vi "image2slopes2phase.vi"(5 "Haso configuration file":path=path "C:/Program Files (x86)/Imagine Optic/Configuration Files/HASO3_first_7364.dat", 7 "Filter":u8[](array[numeric]), 8 "error in (no error)":errorcluster, 9 "Image in":refnum<class "Image.lvclass">, 10 "Phase in":refnum<class "Phase.lvclass">, 11 "HasoSlopes in":refnum<class "HasoSlopes.lvclass">) -> (0 "error out":errorcluster, 1 "Image out":refnum<class "Image.lvclass">, 2 "Phase out":refnum<class "Phase.lvclass">, 3 "HasoSlopes out":refnum<class "HasoSlopes.lvclass">)   [LabVIEW 2018]
uses:
  <userlib>/WaveKit.lib/Classes/Phase/Phase.lvclass
  <userlib>/WaveKit.lib/Controls/HasoSlopes.lvclass
  <userlib>/WaveKit.lib/Classes/Image/Image.lvclass
  <userlib>/WaveKit.lib/Controls/WavefrontReconstructionMode.ctl
  <userlib>/WaveKit.lib/Classes/HasoEngine/HasoEngine.lvclass
  <userlib>/WaveKit.lib/Controls/SlopesEngineSetup.ctl
  <userlib>/WaveKit.lib/Controls/Point2D.ctl
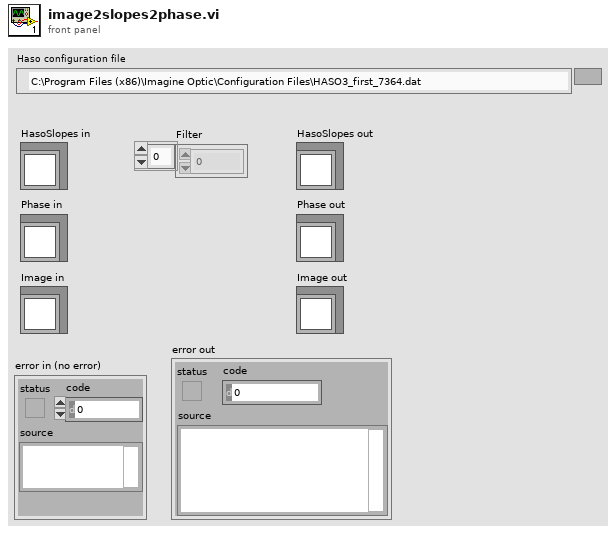
[diagram p1: front panel]
types:
  T1 = typedef "SlopesEngineSetup.ctl" = cluster{"Start sub-aperture":T2, "Pupil average":dbl}
  T2 = typedef "Point2D.ctl" = cluster{"X":u32, "Y":u32}
  T3 = typedef "WavefrontReconstructionMode.ctl" = enum16{"None", "Modal_Legendre", "Modal_Zernike", "Zonal", "Modal_Zonal_Zernike", "Modal_Zonal_Legendre"}
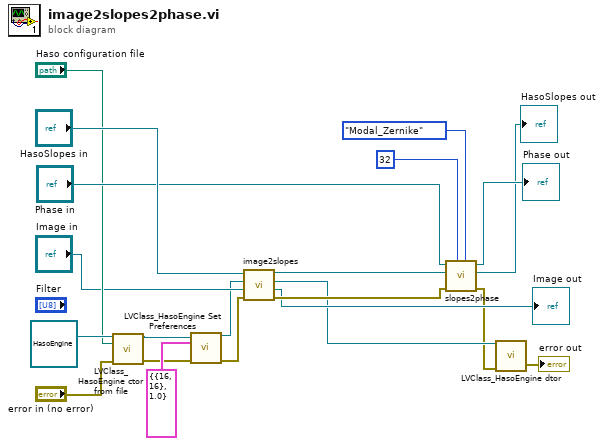
[diagram p0: block diagram]
diagram:
  n1 = call <userlib>:"LVClass_HasoEngine ctor from file.vi"("HasoEngine in"=refnum<class "HasoEngine.lvclass"> refnum, "Configuration file path"="Haso configuration file", "error in (no error)"="error in (no error)") -> ("HasoEngine out"=w1:refnum<class "HasoEngine.lvclass">, "error out"=w2:errorcluster)  [unwired: 11 in]
  n2 = call <userlib>:"LVClass_HasoEngine Set Preferences.vi"("HasoEngine in"=w1, "Slopes_HasoEngine_Setup"=T1 {"Start sub-aperture"={"X"=16, "Y"=16}, "Pupil average"=1.0}, "error in (no error)"=w2) -> ("HasoEngine out"=w4:refnum<class "HasoEngine.lvclass">, "error out"=w3:errorcluster)  [unwired: 11 in]
  n3 = call "image2slopes.vi"("error in (no error)"=w3, "Image in"="Image in", "HasoEngine in"=w4, "HasoSlopes in"="HasoSlopes in") -> ("error out"=w14:errorcluster, "Image out"=→"Image out":refnum<class "Image.lvclass">, "HasoEngine out"=w8:refnum<class "HasoEngine.lvclass">, "HasoSlopes out"=w19:refnum<class "HasoSlopes.lvclass">)  [unwired: 4 in]
  n4 = call "slopes2phase.vi"("TypePhase"=WavefrontReconstructionMode."Modal_Zernike", "Number of coefficients"=u8 32, "error in (no error)"=w14, "HasoSlopes in"=w19, "Phase in"="Phase in") -> ("error out"=w7:errorcluster, "HasoSlopes out"=→"HasoSlopes out":refnum<class "HasoSlopes.lvclass">, "Phase out"=→"Phase out":refnum<class "Phase.lvclass">)  [unwired: 4 in]
  n5 = call <userlib>:"LVClass_HasoEngine dtor.vi"("HasoEngine in"=w8, "error in (no error)"=w7) -> ("error out"=→"error out":errorcluster)  [unwired: 12 in, 1 out]
